vi "Caller.vi"(5 "Initialize-Error Passback":refnum<notifier>, 7 "Events Passback":refnum<notifier>, 9 "Stopped Event":refnum<user-event>, 10 "Launch":refnum<notifier>, 11 "Actor in":refnum<class "Copy of Actor.lvclass">) -> ()   [LabVIEW 2018, in "Copy of Actor.lvclass"]
uses:
  Copy of Actor.lvclass
  Event-References.ctl
  Stop.ctl
  Launched.ctl
  Some Request.ctl
  Some Response.ctl
  Stopped.ctl
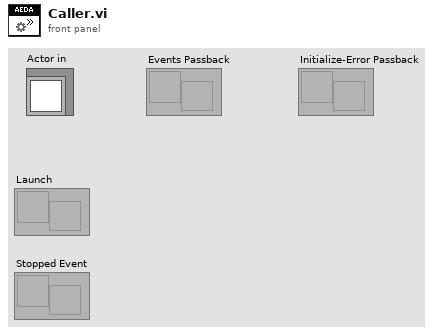
[diagram p1: front panel]
types:
  T1 = typedef "Copy of Actor.lvclass/Stopped.ctl" = cluster{"Final State":refnum<class "Copy of Actor.lvclass">, "Final Error":errorcluster}
  T2 = typedef "Copy of Actor.lvclass/Event-References.ctl" = cluster{"Stop":refnum<user-event>, "Launched":refnum<user-event>, "Some Request":refnum<user-event>}
  T3 = typedef "Copy of Actor.lvclass/Event-Registrations.ctl" = cluster{"Stop":refnum<event-registration>}
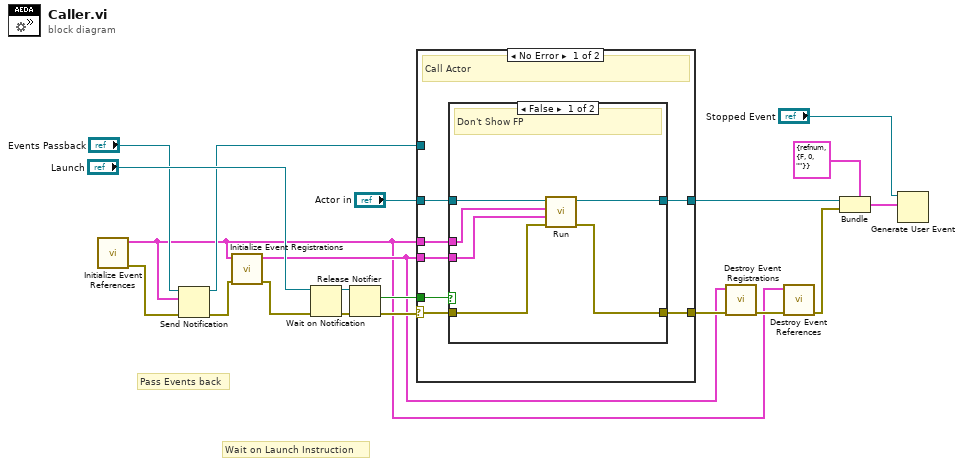
[diagram p0: block diagram]
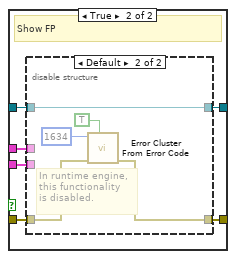
[diagram p2: hidden frame]
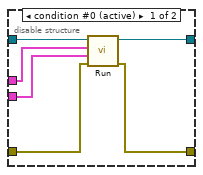
[diagram p3: hidden frame]
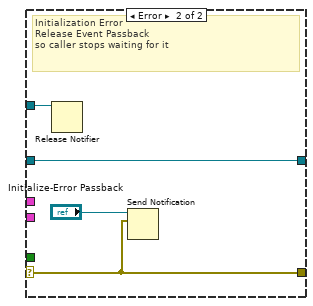
[diagram p4: hidden frame]
diagram:
  # "Wait on Launch Instruction"
  # "Pass Events back"
  n1 = call "Initialize Event References.vi"() -> ("error out"=w8:errorcluster, "Event-References"=w4:T2)  [unwired: 10 in]
  n2 = Send Notification(notification=w4, notifier="Events Passback", error in (no error)=w8) -> (notifier out=w9:refnum<notifier>, error out=w7:errorcluster)
  n3 = call "Initialize Event Registrations.vi"("error in (no error)"=w7, "Events-References"=w4) -> ("error out"=w6:errorcluster, "Event-Registrations"=w5:T3)  [unwired: 8 in]
  n4 = Wait on Notification(notifier="Launch", error in (no error)=w6) -> (notifier out=w20:refnum<notifier>, error out=w19:errorcluster)  [unwired: 2 in, 2 out]
  n5 = Release Notifier(notifier=w20, error in (no error)=w19) -> (last notification=w17:bool, error out=w18:errorcluster)  [unwired: 1 in, 1 out]
  n6 = case shown="No Error" w18 {
    selector: w18 -> [w23 w53]
    tunnel: "Actor in" -> [w27 w54]
    tunnel: w9 -> [_ w52]
    tunnel: [w26 w53] -> w16
    tunnel: [w25 w54] -> w1
    tunnel: w17 -> [w24 _]
    tunnel: w5 -> [w21 _]
    tunnel: w4 -> [w22 _]
    frame No Error {
      # "Call Actor"
      n7 = case shown="False" w24 {
        tunnel: w27 -> [w33 w38]
        tunnel: [w32 w36] -> w26
        tunnel: [w31 w37] -> w25
        tunnel: w23 -> [w30 w39]
        tunnel: w22 -> [w29 w35]
        tunnel: w21 -> [w28 w34]
        frame False {
          # "Don't Show FP"
          n8 = call-dynamic "Run.vi"("error in"=w30, "Actor-Event-Registrations"=w28, "Actor-Events"=w29, "Actor in"=w33) -> ("error out"=w32:errorcluster, "Actor out"=w31:refnum<class "Copy of Actor.lvclass">)  [unwired: 6 in]
        }
        frame True {
          # "Show FP"
          n9 = disable-structure shown="Default" {
            disable-tunnel: [w43 w49] -> w36
            disable-tunnel: [w42 w50] -> w37
            disable-tunnel: w38 -> [w45 w50]
            disable-tunnel: w39 -> [w44 w48]
            disable-tunnel: w35 -> [w41 _]
            disable-tunnel: w34 -> [w40 _]
            frame condition #0 (active) {
              n10 = call-dynamic "Run.vi"("error in"=w44, "Actor-Event-Registrations"=w40, "Actor-Events"=w41, "Actor in"=w45) -> ("error out"=w43:errorcluster, "Actor out"=w42:refnum<class "Copy of Actor.lvclass">)  [unwired: 6 in]
            }
            frame condition #1 {
              # "In runtime engine,\nthis functionality\nis disabled."
              n11 = call <vilib>:"Error Cluster From Error Code.vi"("show call chain? (False)"=TRUE, "error in (no error)"=w48, "error code (0)"=1634) -> ("error out"=w49:errorcluster)  [unwired: 6 in]
            }
          }
        }
      }
    }
    frame Error {
      # "Initialization Error\nRelease Event Passback\nso caller stops waiting for it"
      n12 = Release Notifier(notifier=w52) -> ()  [unwired: 2 in, 3 out]
      n13 = Send Notification(notification=w53, notifier="Initialize-Error Passback") -> ()  [unwired: 1 in, 2 out]
    }
  }
  n14 = call "Destroy Event Registrations.vi"("error in (no error)"=w16, "Event-Registrations"=w5) -> ("error out"=w15:errorcluster)  [unwired: 9 in]
  n15 = call "Destroy Event References.vi"("error in (no error)"=w15, "Event-References"=w4) -> ("error out"=w2:errorcluster)  [unwired: 9 in]
  n16 = Bundle(cluster=T1 {"Final State"=refnum, "Final Error"={"status"=FALSE, "code"=0, "source"=""}} ("event data"), "Final State"=w1, "Final Error"=w2) -> (w13:T1)
  n17 = Generate User Event(user event="Stopped Event", event data cluster=w13) -> ()  [unwired: 2 in, 2 out]
